vi "Read Errors count.vi"(11 "Test Suite Result In":T1) -> (1 "Error count string":string, 2 "Errors count":i32, 3 "Test Suite Result Out":T1)   [LabVIEW 2020, in "Test Suite Result.lvlib"]
uses:
  Test Suite Result.lvlib
  Assertion Result/Public/TypeDefs/Status.ctl
  Assertion Result/Assertion Result.lvlib
  Assertion Result/Public/TypeDefs/Assertion Type.ctl
  Assertion Result/Assertion Result.ctl
  Method Result/Method Result.ctl
  Method Result/Method Result.lvlib
  Case Result/Test Case Result.ctl
  Case Result/Test Case Result.lvlib
  Test Suite Result.ctl
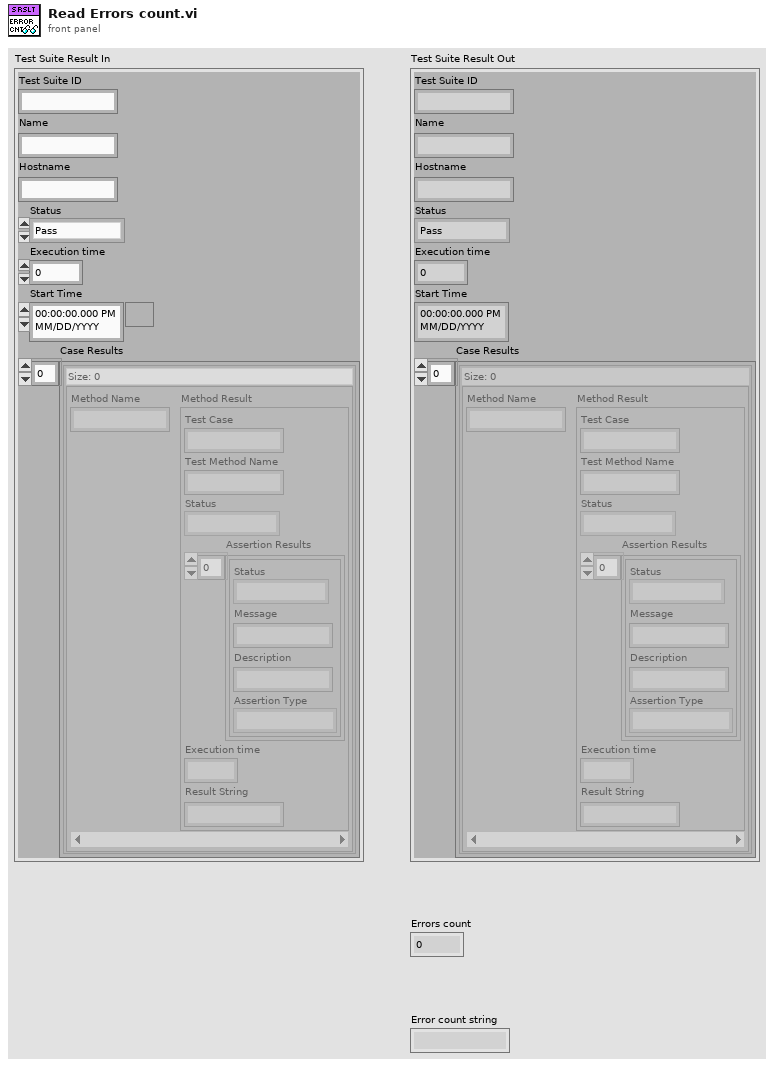
[diagram p1: front panel]
types:
  T1 = typedef "Test Suite Result.lvlib/Test Suite Result.ctl" = cluster{"Test Suite ID":string, "Name":string, "Hostname":string, "Status":T2, "Execution time":dbl, "Start Time":timestamp, "Case Results":T3[]}
  T2 = typedef "Assertion Result.lvlib/Status.ctl" = enum16{"Pass", "Fail", "Error", "Skipped", "Setup Error", "Broken", "Teardown Error"}
  T3 = typedef "Test Case Result.lvlib/Test Case Result.ctl" = map{string, T4}
  T4 = typedef "Method Result.lvlib/Method Result.ctl" = cluster{"Test Case":string, "Test Method Name":string, "Status":T2, "Assertion Results":T5[], "Execution time":dbl, "Result String":string}
  T5 = typedef "Assertion Result.lvlib/Assertion Result.ctl" = cluster{"Status":T2, "Message":string, "Description":string, "Assertion Type":T6}
  T6 = typedef "Assertion Result.lvlib/Assertion Type.ctl" = enum16{"None", "Pass", "Fail", "Skip", "Pass if Equal", "Fail if Equal", "Pass if Error", "Fail if Error", "Pass if", "Fail if"}
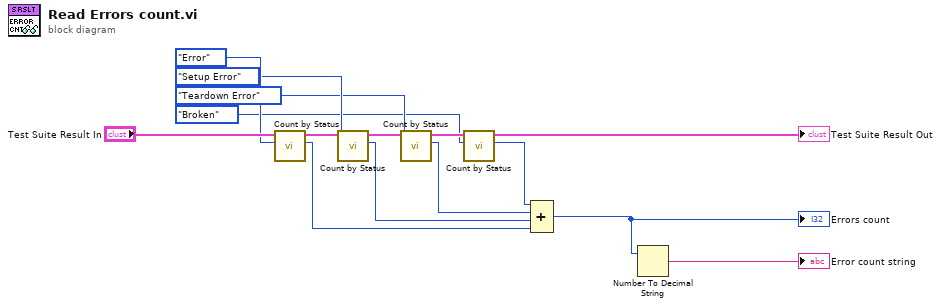
[diagram p0: block diagram]
diagram:
  n1 = call "Count by Status.vi"("Status"=Status."Error", "Test Suite Result in"="Test Suite Result In") -> ("Count"=w1:i32, "Test Suite Result out"=w14:T1)  [unwired: 8 in]
  n2 = call "Count by Status.vi"("Status"=Status."Setup Error", "Test Suite Result in"=w14) -> ("Count"=w2:i32, "Test Suite Result out"=w13:T1)  [unwired: 8 in]
  n3 = call "Count by Status.vi"("Status"=Status."Teardown Error", "Test Suite Result in"=w13) -> ("Count"=w3:i32, "Test Suite Result out"=w8:T1)  [unwired: 8 in]
  n4 = call "Count by Status.vi"("Status"=Status."Broken", "Test Suite Result in"=w8) -> ("Count"=w4:i32, "Test Suite Result out"=→"Test Suite Result Out":T1)  [unwired: 8 in]
  n5 = Compound Arithmetic op=ADD(w4, w3, w2, w1) -> (w5:i32)
  "Errors count" <- w5
  n6 = Number To Decimal String(number=w5) -> (decimal integer string=→"Error count string":string)  [unwired: 1 in]
